vi "Init AI Channel.vi"(8 "error in":errorcluster, 9 "Channel Configuration":T1={"Channel#"=0, "Measurement Type"=0, "Position_LVDT_Properties"={"Minimum Value"=-0.1, "Maximum Value"=0.1, "Excitation Source"=10200, "Excitation Wire Mode"=4, "Excitation Frequency"=2500.0, "Excitation Value"=1.0, "Units"=10219, "Sensitivity"=50.0, "Sensitivity Units"=12506, "Excitation Sense"=16095}, "Position_RVDT_Properties"={"Minimum Value"=-70.0, "Maximum Value"=70.0, "Excitation Source"=10200, "Excitation Wire Mode"=4, "Excitation Frequency"=2500.0, "Excitation Value"=1.0, "Units"=10146, "Sensitivity"=50.0, "Sensitivity Units"=12507, "Excitation Sense"=16095}} {"Position_RVDT_Properties"."Sensitivity Units" items=["mVolts/Volt/Degree"=12507, "mVolts/Volt/Radian"=12508]; "Position_RVDT_Properties"."Units" items=["Degrees"=10146, "Radians"=10273, "From Custom Scale"=10065]; "Position_RVDT_Properties"."Excitation Sense" items=["Local"=16095, "Remote"=16096]; "Position_RVDT_Properties"."Excitation Source" items=["Internal"=10200, "External"=10167, "None"=10230]; "Position_RVDT_Properties"."Excitation Wire Mode" items=["4-Wire"=4, "5-Wire"=5, "6-Wire"=6]; "Position_LVDT_Properties"."Excitation Sense" items=["Local"=16095, "Remote"=16096]; "Position_LVDT_Properties"."Excitation Source" items=["Internal"=10200, "External"=10167, "None"=10230]; "Position_LVDT_Properties"."Excitation Wire Mode" items=["4-Wire"=4, "5-Wire"=5, "6-Wire"=6]; "Position_LVDT_Properties"."Units" items=["Meters"=10219, "Inches"=10379, "From Custom Scale"=10065]; "Position_LVDT_Properties"."Sensitivity Units" items=["mVolts/Volt/mMeter"=12506, "mVolts/Volt/0.001 Inch"=12505]; "Measurement Type" items=["Position LVDT", "Position RVDT"]}, 10 "Device Name":string, 11 "task in":refnum<k21>) -> (0 "error out":errorcluster, 3 "task out":refnum<k21>)   [LabVIEW 2020, in "NI PXIe-4340 Engine.lvlib"]
uses:
  NI PXIe-4340 Engine.lvlib
  Shared/Channel Configuration.ctl
  Shared/Position_LVDT_Properties.ctl
  Shared/Position_RVDT_Properties.ctl
  Shared/NI PXIe-4340 Shared.lvlib
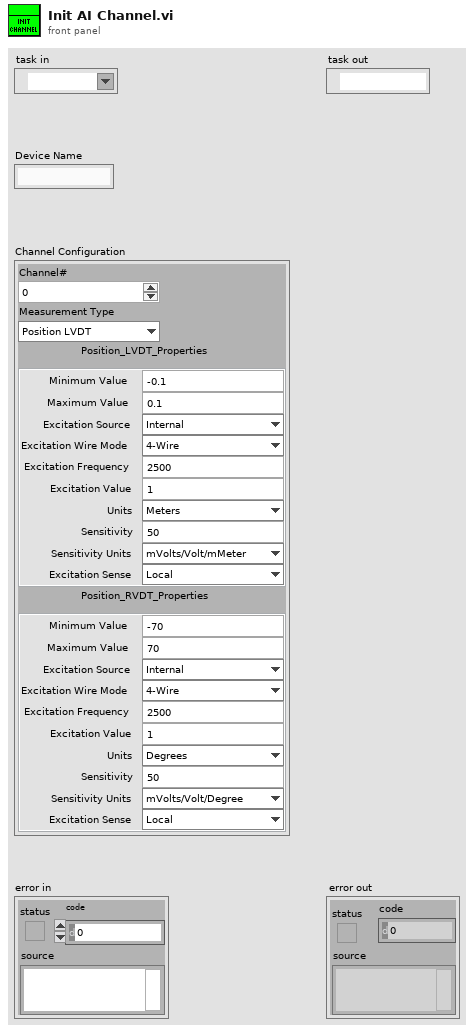
[diagram p1: front panel]
types:
  T1 = typedef "NI PXIe-4340 Shared.lvlib/Channel Configuration.ctl" = cluster{"Channel#":i32, "Measurement Type":i32, "Position_LVDT_Properties":T2, "Position_RVDT_Properties":T3}
  T2 = typedef "NI PXIe-4340 Shared.lvlib/Position_LVDT_Properties.ctl" = cluster{"Minimum Value":dbl, "Maximum Value":dbl, "Excitation Source":i32, "Excitation Wire Mode":i32, "Excitation Frequency":dbl, "Excitation Value":dbl, "Units":i32, "Sensitivity":dbl, "Sensitivity Units":i32, "Excitation Sense":i32}
  T3 = typedef "NI PXIe-4340 Shared.lvlib/Position_RVDT_Properties.ctl" = cluster{"Minimum Value":dbl, "Maximum Value":dbl, "Excitation Source":i32, "Excitation Wire Mode":i32, "Excitation Frequency":dbl, "Excitation Value":dbl, "Units":i32, "Sensitivity":dbl, "Sensitivity Units":i32, "Excitation Sense":i32}
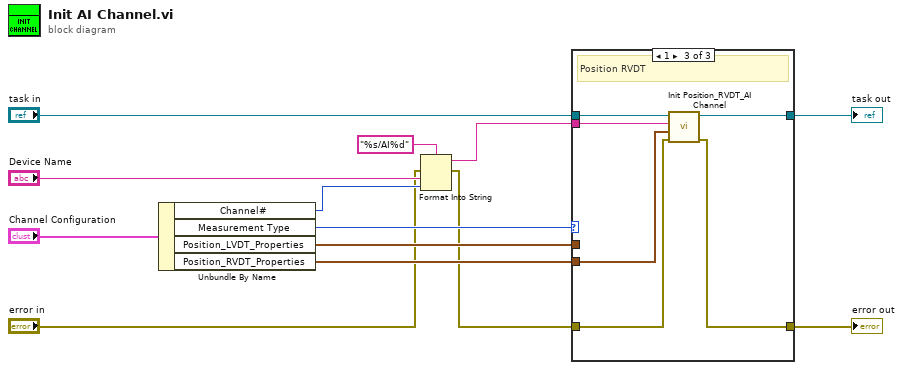
[diagram p0: block diagram]
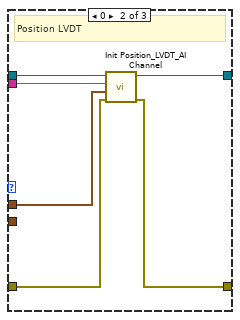
[diagram p3: hidden frame]
diagram:
  n1 = Unbundle By Name("Channel Configuration") -> ("Channel#"=w3:i32, "Measurement Type"=w10:i32, "Position_LVDT_Properties"=w9:T2, "Position_RVDT_Properties"=w8:T3)
  n2 = Format Into String(format string="%s/AI%d", error in="error in", "Device Name", w3) -> (resulting string=w11:string, error out=w1:errorcluster)  [unwired: 1 in]
  n3 = case shown="1" w10 {
    tunnel: "task in" -> [w14 w21 w27]
    tunnel: w11 -> [_ w20 w26]
    tunnel: w9 -> [_ w19 _]
    tunnel: w1 -> [w15 w18 w25]
    tunnel: w8 -> [_ _ w24]
    tunnel: [w15 w17 w23] -> w7
    tunnel: [w14 w16 w22] -> w4
    frame Default {
    }
    frame 0 {
      # "Position LVDT"
      n4 = call "Init Position_LVDT_AI Channel.vi"("error in"=w18, "Position_LVDT_Properties"=w19, "physical channel"=w20, "task in"=w21) -> ("error out"=w17:errorcluster, "task out"=w16:refnum<k21>)  [unwired: 6 in]
    }
    frame 1 {
      # "Position RVDT"
      n5 = call "Init Position_RVDT_AI Channel.vi"("error in"=w25, "Position_RVDT_Properties"=w24, "physical channels"=w26, "task in"=w27) -> ("error out"=w23:errorcluster, "task out"=w22:refnum<k21>)  [unwired: 6 in]
    }
  }
  "error out" <- w7
  "task out" <- w4
